vi "Number to BCD.vi"(11 "Number":u8) -> (3 "BCD":u8 format="%x")   [LabVIEW 2024]
doc: "This VI converts an U32 to Binary Coded Decimal. Each digit can take up to 4 bits, so two digits can fit in to a single U8. This can be optionally toggled"
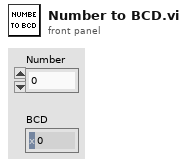
[diagram p1: front panel]
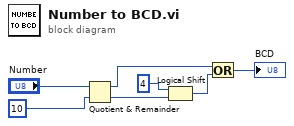
[diagram p0: block diagram]
diagram:
  n1 = Quotient & Remainder(x="Number", y=u8 10) -> (x-y*floor(x/y)=w1:u8, floor(x/y)=w3:u8)
  n2 = Logical Shift(y=u8 4, x=w3) -> (x << y=w2:u8)
  n3 = Or(x=w1, y=w2) -> (x .or. y?=→"BCD":u8)
